vi "RunService_CLIWrapper.vi"(11 "Inputs":string[](array[string])) -> (2 "Output/Failure":string, 3 "CLI Process Return Code":i32)   [LabVIEW 2019]
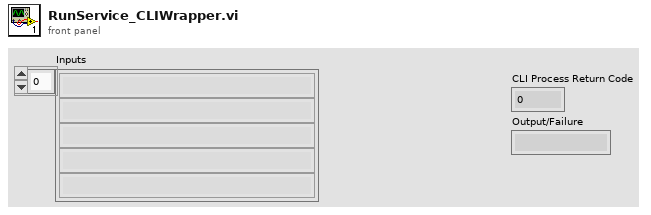
[diagram p1: front panel]
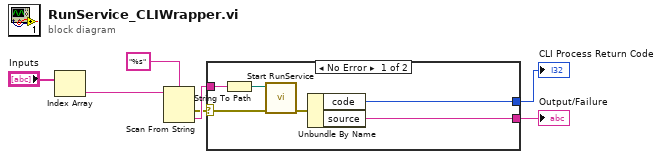
[diagram p0: block diagram]
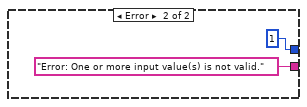
[diagram p2: hidden frame]
diagram:
  n1 = Index Array "Index Array"(array="Inputs") -> (element=w4:string)  [unwired: 1 in]
  n2 = Scan From String(format string="%s", input string=w4) -> (error out=w1:errorcluster, output 1=w5:string)  [unwired: 3 in, 2 out]
  n3 = case shown="No Error" w1 {
    selector: w1 -> [w9 _]
    tunnel: [w10 1] -> w2
    tunnel: [w11 "Error: One or more input value(s) is not valid."] -> w3
    tunnel: w5 -> [w13 _]
    frame No Error {
      n4 = String To Path(string=w13) -> (path=w12:path)
      n5 = call "Start RunService.vi"("error in (no error)"=w9, "project folder"=w12) -> ("error out"=w8:errorcluster)  [unwired: 8 in, 1 out]
      n6 = Unbundle By Name(w8) -> ("code"=w10:i32, "source"=w11:string)
    }
    frame Error {
    }
  }
  "CLI Process Return Code" <- w2
  "Output/Failure" <- w3
